vi "Check NewStateNotify is Registered.vi"(8 "error in (no error)":errorcluster, 11 "CSM-Helper in":refnum<class "CSM-Helper.lvclass">) -> (0 "error out":errorcluster, 2 "NewStateNotify Registed":bool, 3 "CSM-Helper out":refnum<class "CSM-Helper.lvclass">)   [LabVIEW 2017, in "CSM-Helper.lvclass"]
doc: "### Check NewStateNotify is Registered.vi\n\n-- <b>Controls</b> --\n- <b>CSM-Helper in</b>: CSMHelper input\n\n-- <b>Indicators</b> --\n- <b>NewStateNotify Registered</b>:\n- <b>CSM-Helper out</b>: CSMHelper output"
uses:
  CSM-Helper.lvclass
  CSM-Helper.lvclass/CSM-Helper.ctl
  Properties/Read Event Structure Ref.vi
  _Shared/CSM Shared.lvlib
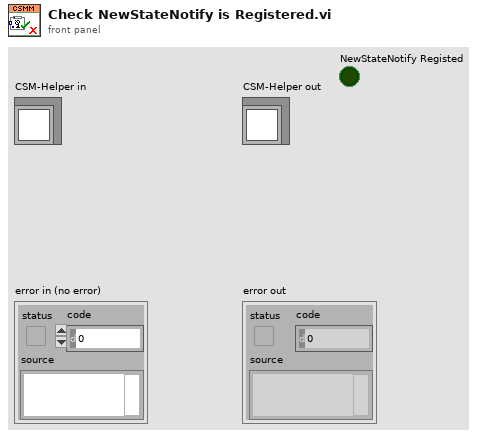
[diagram p1: front panel]
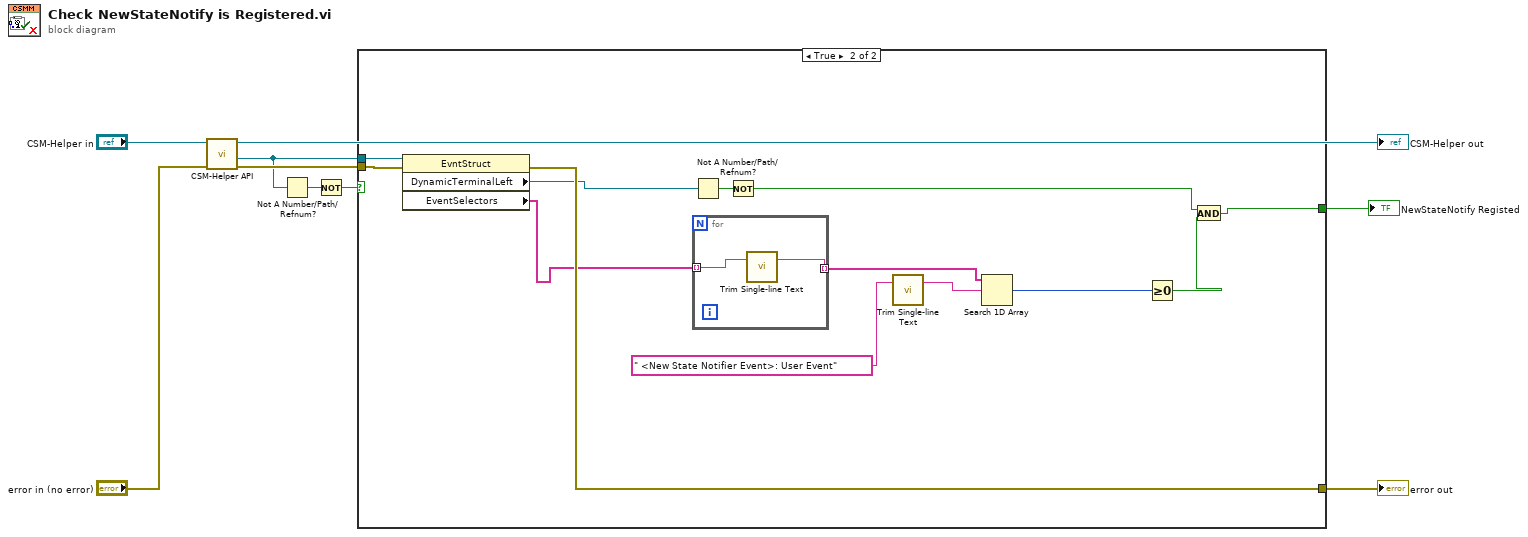
[diagram p0: block diagram]
diagram:
  n1 = call-poly "CSM-Helper API.vi"("error in (no error)"="error in (no error)", "CSM-Helper in"="CSM-Helper in") -> ("error out"=w6:errorcluster, "Event Structure"=w4:refnum<vi>, "CSM-Helper out"=→"CSM-Helper out":refnum<class "CSM-Helper.lvclass">)  [unwired: 7 in]
  n2 = Not A Number/Path/Refnum?(number/path/refnum=w4) -> (NaN/Path/Refnum?=w3:bool)
  n3 = Not(x=w3) -> (.not. x?=w1:bool)
  n4 = case shown="True" w1 {
    tunnel: w6 -> [w10 w23]
    tunnel: [w10 w22] -> w5
    tunnel: w4 -> [_ w21]
    tunnel: [_ w12] -> w2
    frame False {
    }
    frame True {
      n5 = property class="EvntStruct"(reference=w21, error in=w23) -> (error out=w22:errorcluster, "DynamicTerminalLeft"=w20:refnum<vi>, "EventSelectors"=w15:string[])  [unwired: 1 out]
      n6 = Not A Number/Path/Refnum?(number/path/refnum=w20) -> (NaN/Path/Refnum?=w14:bool)
      n7 = for {
        tunnel: [w24] -> w16 mode=indexing
        tunnel: w15 -> [w25] mode=indexing
        n8 = call "Trim Single-line Text.vi"("single-line text"=w25) -> ("trimed text"=w24:string)  [unwired: 2 in]
      }
      n9 = Not(x=w14) -> (.not. x?=w11:bool)
      n10 = call "Trim Single-line Text.vi"("single-line text"=" <New State Notifier Event>: User Event" ("element")) -> ("trimed text"=w17:string)  [unwired: 2 in]
      n11 = Search 1D Array(1D array=w16, element=w17) -> (index of element=w19:i32)  [unwired: 1 in]
      n12 = Greater Or Equal To 0?(x=w19) -> (x >= 0?=w13:bool)
      n13 = And(x=w11, y=w13) -> (x .and. y?=w12:bool)
    }
  }
  "error out" <- w5
  "NewStateNotify Registed" <- w2
